vi "Main.vi"() -> ()   [LabVIEW 2012]
uses:
  <vilib>/Platform/TimedLoop/XDataNode/timing_clust.ctl
  <vilib>/Platform/TimedLoop/XDataNode/nitl_modes.ctl
  <vilib>/Platform/TimedLoop/XDataNode/wakeup.ctl
  <vilib>/Platform/TimedLoop/XDataNode/XDataNode.xnode
  <vilib>/Platform/TimedLoop/XDataNode/XDNodeRunTimeDep.lvlib
panel:
  in  "Tab Control":enum32{"IMU", "Control", "Status", "Errors"}(tab)
  in  "IMU VISA":refnum<visa-resource-name>="ASRL1::INSTR"
  in  "PID gains":T1={"proportional gain (Kc)"=30.0, "integral time (Ti, min)"=0.0, "derivative time (Td, min)"=0.1} {"derivative time (Td, min)" format="%.3f"; "integral time (Ti, min)" format="%.3f"; "proportional gain (Kc)" format="%.3f"}
  in  "Setpoint":dbl(knob) scale=-0.5..0.5
  out "States":dbl[](array[numeric])
  in  "Parameters":T2={"Limit"=10.0, "Control Dead Band"=20.0, "Error Dead Band"=20.0}
  out "Read Loop Count":i32
  out "Received array Size":i32
  out "Processing Loop Count":i32
  out "Command to Serial":string
  out "timed out?":bool
  out "Serial Settings:Number of Bytes at Serial Port":u32
  out "Byte Count":u32
  out "IMU Rean Error":errorcluster
  in  "Error In":errorcluster
  out "RoboteQ Error":errorcluster
  out "Error Out":errorcluster
  in  "stop?":bool
  out "Roll":dbl(knob) scale=-20.0..20.0
  out "Status":string="Kill"
  in  "Kill":bool
  in  "Enable":bool
  out "Top Motor Effort":dbl(knob) scale=-1000.0..1000.0
  out "Bottom Motor Effort":dbl(knob) scale=-1000.0..1000.0
  in  "Mode":T3(ring)
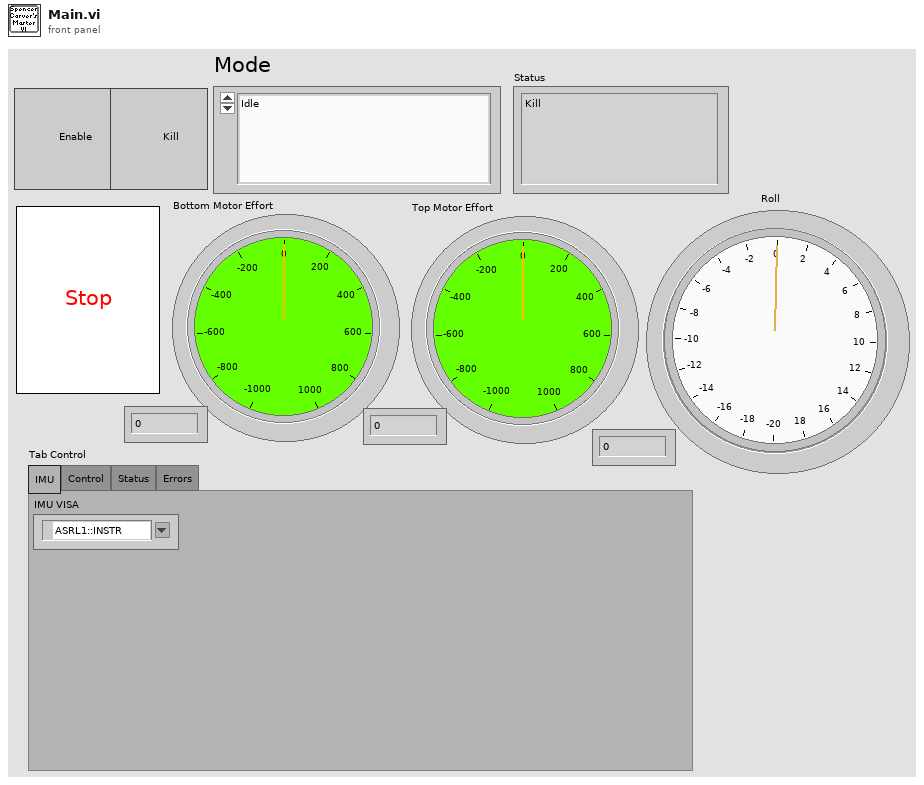
[diagram p1: front panel]
types:
  T1 = cluster{"proportional gain (Kc)":dbl, "integral time (Ti, min)":dbl, "derivative time (Td, min)":dbl}
  T2 = cluster{"Limit":dbl, "Control Dead Band":dbl, "Error Dead Band":dbl}
  T3 = enum16{"Idle", "Linear Balance", "Proportional Balance", "PID Balance", "Emergency"}
  T4 = typedef "901x DMA FPGA Reference.ctl" = refnum<k20>
  T5 = typedef "XDNodeRunTimeDep.lvlib/timing_clust.ctl" = cluster{"Expected End [f-1]":u64, "Actual End [f-1]":u64, "Finished Late? [f-1]":bool, "Expected End [i-1]":u64, "Actual End [i-1]":u64, "Finished Late? [i-1]":bool, "Expected Start [i]":u64, "Actual Start [i]":u64, "Expected Start [f]":u64, "Actual Start [f]":u64, "Source Name":string, "Structure Name":string, "Period":i64, "Deadline":i64, "Offset":i64, "Start":i64, "Priority":i32, "Timeout":i32, "Mode":T6, "Wakeup Reason":T7, "Error":errorcluster, "Source Type":string, "Secondary Source Type":string, "Global End Time":u64, "Global Start Time":u64, "Frame Duration":u64, "Iteration Duration":u64, "Assigned CPU":i32, "I/O Scan Engine Mode":u32}
  T6 = typedef "XDNodeRunTimeDep.lvlib/nitl_modes.ctl" = enum32{"No Change", "Process missed periods, maintain original phase", "Discard missed periods, maintain original phase", "Process missed periods, ignore original phase", "Discard missed periods, ignore original phase"}
  T7 = typedef "XDNodeRunTimeDep.lvlib/wakeup.ctl" = enum32{"Normal", "Aborted", "Asynchronous wakeup", "Timing source error", "Timed loop error", "Timeout"}
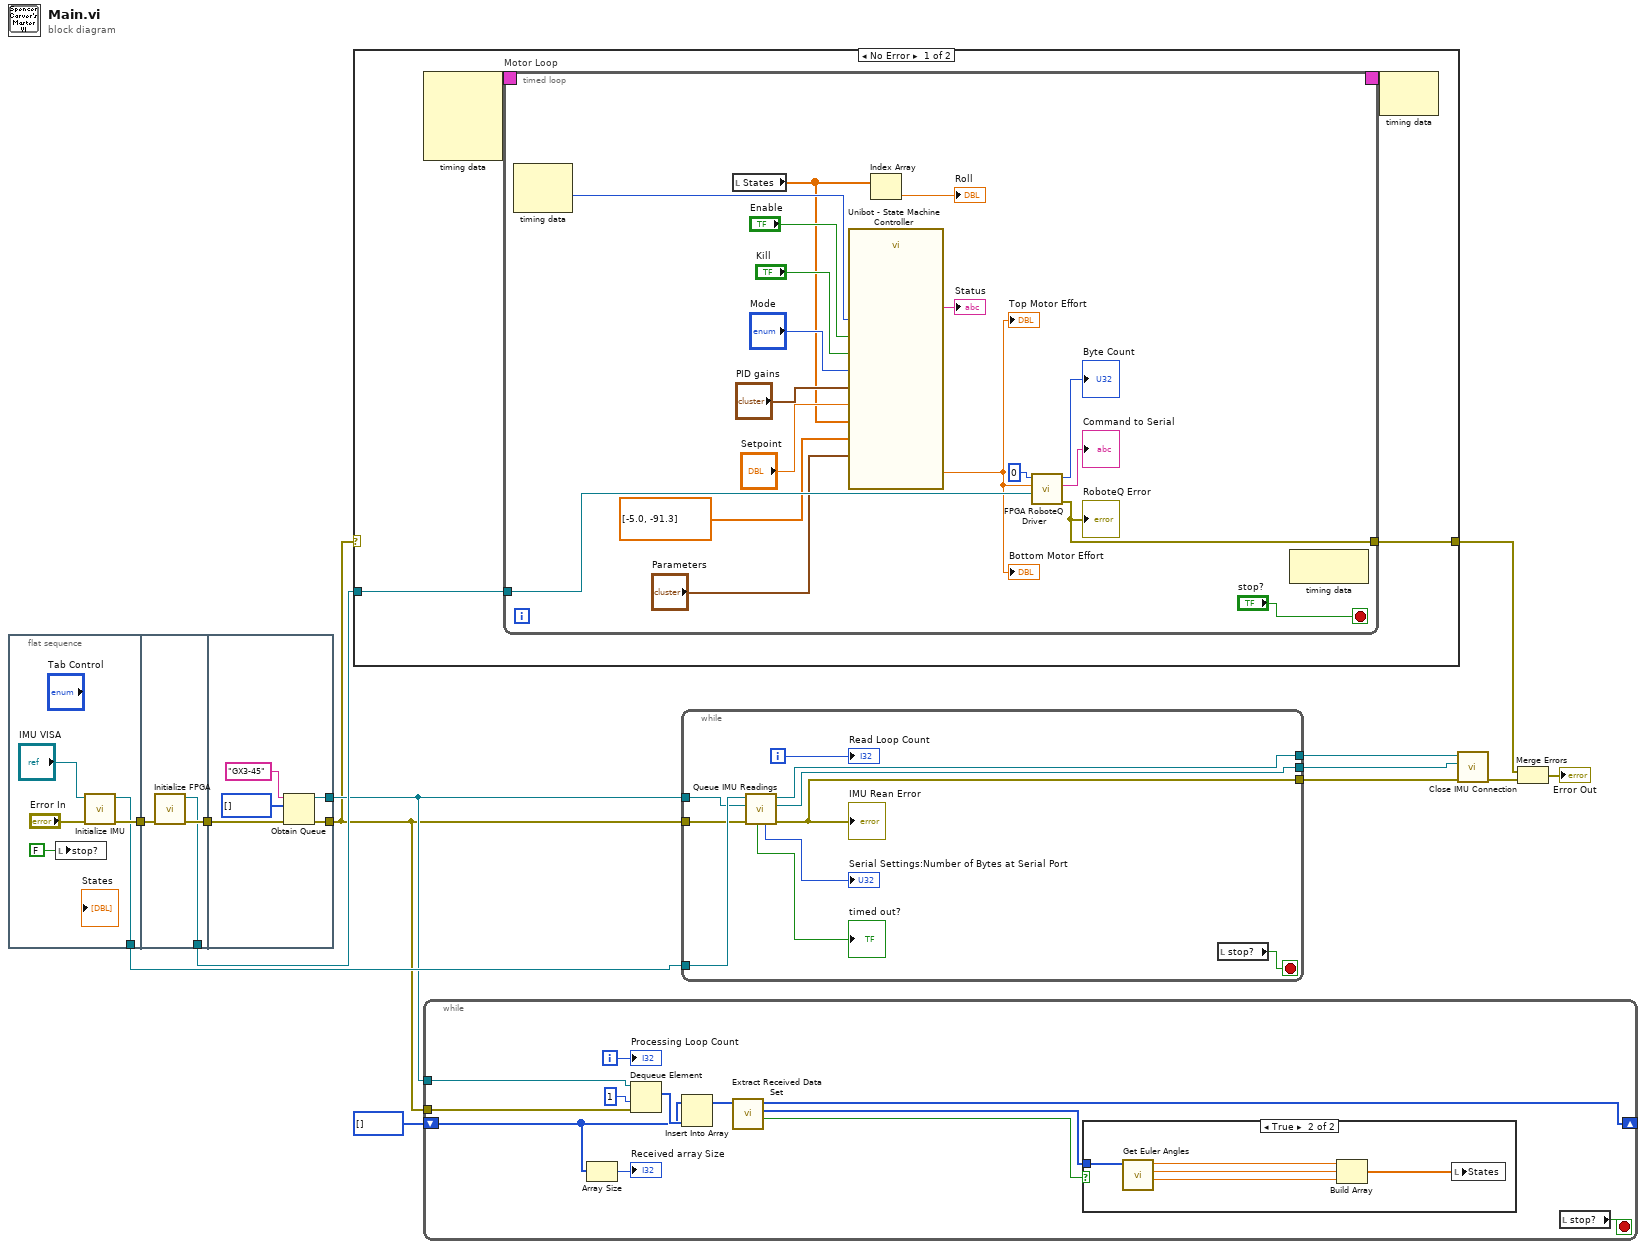
[diagram p0: block diagram]
diagram:
  n1 = flat-sequence {
    tunnel: [w16] -> w6
    tunnel: [w15] -> w3
    tunnel: w6 -> [w21]
    tunnel: [w20] -> w5
    tunnel: [w19] -> w4
    tunnel: w5 -> [w24]
    tunnel: [w23] -> w2
    tunnel: [w22] -> w1
    frame #0 {
      n2 = local write "stop?"(FALSE ("stop?")) -> ()
      n3 = call "Initialize IMU.vi"("error in (no error)"="Error In", "IMU VISA"="IMU VISA") -> ("error out"=w16:errorcluster, "VISA resource name out"=w15:refnum<visa-resource-name>)  [unwired: 8 in]
    }
    frame #1 {
      n4 = call "Initialize FPGA.vi"("error in"=w21) -> ("error out"=w20:errorcluster, "FPGA Out"=w19:T4)  [unwired: 9 in]
    }
    frame #2 {
      n5 = Obtain Queue(name (unnamed)="GX3-45", element data type=u8[] [] ("unsigned byte array"), error in (no error)=w24) -> (queue out=w23:refnum<queue>, error out=w22:errorcluster)  [unwired: 2 in, 1 out]
    }
  }
  n6 = case shown="No Error" w1 {
    selector: w1 -> [_ w54]
    tunnel: [w28 w54] -> w9
    tunnel: w4 -> [w27 _]
    frame No Error {
      n7 = node-c288() -> (w30:T5)  [unwired: 4 in]
      n8 = timed-loop "Motor Loop" {
        timing: w30 -> [_]
        timing-out: [_] -> w29
        tunnel: w27 -> [w48]
        tunnel: [w36] -> w28
        stop <- "stop?" stop-if-true
        n9 = node-c288() -> (w44:i64)  [unwired: 1 in, 1 out]
        n10 = local read "States"() -> (w38:dbl[])
        n11 = call "Unibot - State Machine Controller.vi"("dt (s)"=w44, "Parameters"="Parameters", "Up Optimal Gain"=dbl[] [-5.0, -91.3], "Mode"="Mode", "Setpoint"="Setpoint", "Enable"="Enable", "Kill"="Kill", "PID gains"="PID gains", "States"=w38) -> ("Status"=→"Status":string, "Control Effort"=w33:dbl)  [unwired: 1 in]
        "Top Motor Effort" <- w33
        "Bottom Motor Effort" <- w33
        n12 = Index Array(array=w38) -> (element=→"Roll":dbl)  [unwired: 1 in]
        n13 = call "FPGA RoboteQ Driver.vi"("FPGA In"=w48, "Motor 2 Effort"=w33, "Motor 1 Effort"=0) -> ("error out"=w36:errorcluster, "Command to Serial"=→"Command to Serial":string, "Byte Count"=→"Byte Count":u32)  [unwired: 5 in, 1 out]
        "RoboteQ Error" <- w36
        n14 = node-c288() -> ()  [unwired: 1 in, 1 out]
      }
      n15 = node-c288(w29) -> ()  [unwired: 1 out]
    }
    frame Error {
    }
  }
  n16 = while {
    shift-right: [w58] -> _
    shift-left: u8[] [] ("element") -> [w62]
    tunnel: w2 -> [w57]
    tunnel: w1 -> [w56]
    i -> [w65]
    stop <- w55 stop-if-true
    n17 = Array Size(array=w62) -> (size(s)=→"Received array Size":i32)
    n18 = Dequeue Element(queue=w57, timeout in ms (-1)=1, error in (no error)=w56) -> (element=w66:u8[])  [unwired: 3 out]
    n19 = Insert Into Array(array=w62, new element=w66) -> (w64:u8[])  [unwired: 1 in]
    n20 = call "Extract Received Data Set.vi"("Received Array In"=w64) -> ("New Data Set Received"=w60:bool, "Extracted Data Set"=w59:u8[], "Received Array Out"=w58:u8[])  [unwired: 7 in, 1 out]
    n21 = case shown="True" w60 {
      tunnel: w59 -> [_ w71]
      frame False {
      }
      frame True {
        n22 = call "Get Euler Angles.vi"("Received Array"=w71) -> ("Yaw (deg)"=w69:dbl, "Pitch (deg)"=w68:dbl, "Roll (deg)"=w70:dbl)  [unwired: 7 in]
        n23 = Build Array(w70, w68, w69) -> (w67:dbl[])
        n24 = local write "States"(w67) -> ()
      }
    }
    n25 = local read "stop?"() -> (w55:bool)
    "Processing Loop Count" <- w65
  }
  n26 = while {
    tunnel: [w80] -> w10
    tunnel: [w79] -> w11
    tunnel: [w78] -> w7
    tunnel: w3 -> [w75]
    tunnel: w2 -> [w74]
    tunnel: w1 -> [w73]
    i -> [w81]
    stop <- w72 stop-if-true
    n27 = call "Queue IMU Readings.vi"("error in (no error)"=w73, "queue"=w74, "reference"=w75) -> ("error out"=w79:errorcluster, "queue out"=w78:refnum<queue>, "VISA resource name out"=w80:refnum<visa-resource-name>, "Serial Settings:Number of Bytes at Serial Port"=→"Serial Settings:Number of Bytes at Serial Port":u32, "timed out?"=→"timed out?":bool)  [unwired: 4 in]
    "IMU Rean Error" <- w79
    n28 = local read "stop?"() -> (w72:bool)
    "Read Loop Count" <- w81
  }
  n29 = call "Close IMU Connection.vi"("Error In"=w11, "queue"=w7, "VISA resource name"=w10) -> ("error out"=w13:errorcluster)  [unwired: 8 in]
  n30 = Merge Errors(w9, w13) -> (→"Error Out":errorcluster)
